vi "Write Resource Name.vi"(8 "error in (no error)":errorcluster, 10 "Resource Name":string, 11 "CS++DeviceActor in":refnum<class "CS++DeviceActor.lvclass">) -> (0 "error out":errorcluster, 3 "CS++DeviceActor out":refnum<class "CS++DeviceActor.lvclass">)   [LabVIEW 2013, in "CS++DeviceActor.lvlib" / "CS++DeviceActor.lvclass"]
doc: "Write instrument resource name."
uses:
  CS++DeviceActor.lvclass
  CS++DeviceActor.lvclass/CS++DeviceActor.ctl
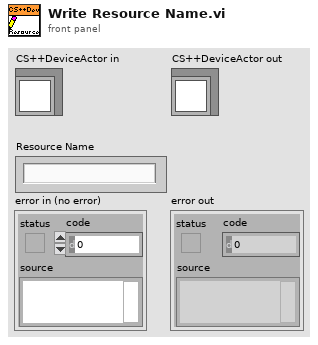
[diagram p1: front panel]
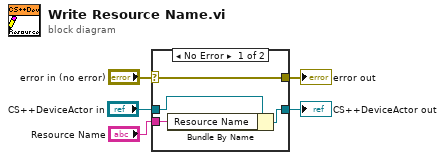
[diagram p0: block diagram]
diagram:
  n1 = case shown="No Error" "error in (no error)" {
    selector: "error in (no error)" -> [w9 w10]
    tunnel: [w9 w10] -> w4
    tunnel: [w7 w11] -> w2
    tunnel: "CS++DeviceActor in" -> [w8 w11]
    tunnel: "Resource Name" -> [w6 _]
    frame No Error {
      n2 = Bundle By Name(cluster=w8, "Resource Name"=w6) -> (w7:refnum<class "CS++DeviceActor.lvclass">)
    }
    frame Error {
    }
  }
  "error out" <- w4
  "CS++DeviceActor out" <- w2
